vi "NetworkPlots.vi"(10 "ControlRefs":T1, 11 "VisualizeData":T2 {"clPmuImpairRptArray"."Synx" format="%#_4g"; "clEvtReportArray"."Synx" format="%#_4g"}) -> ()   [LabVIEW 2014, in "Visualization.lvlib" / "VisualizeNetwork_class.lvclass"]
uses:
  VisualizeNetwork_class.lvclass
  VisializeBase_class/Typedefs/VisualizeData.ctl
  VisializeBase_class/Typedefs/clVisualizeData.ctl
  Modules/EventPlugins/EventPluginBaseClass/TypeDefs/clEvtReportArray.ctl
  Modules/EventPlugins/EventPluginBaseClass/TypeDefs/clEvtReport.ctl
  Modules/EventPlugins/EventPluginBaseClass/TypeDefs/dblEvtSignalArray.ctl
  Modules/NetworkImpairmentModule/PublicAPI/Arguments/Broadcasts/dblNetworkTime.ctl
  Modules/NetworkImpairmentModule/PublicAPI/Arguments/Broadcasts/dblPktLoss.ctl
  Modules/FlagImpairModule/PublicAPI/Arguments/Broadcasts/ui32FlagImpairmentArray.ctl
  Modules/EventPlugins/EventPluginBaseClass/EventPluginBaseClass.lvclass
  Modules/NetworkImpairmentModule/NetworkImpairmentModule.lvlib
  Modules/FlagImpairModule/FlagImpairModule.lvlib
  VisializeBase_class/VisualizeBase_class.lvclass
  VisualizeApp_class/VisualizeAppBase_class.lvclass
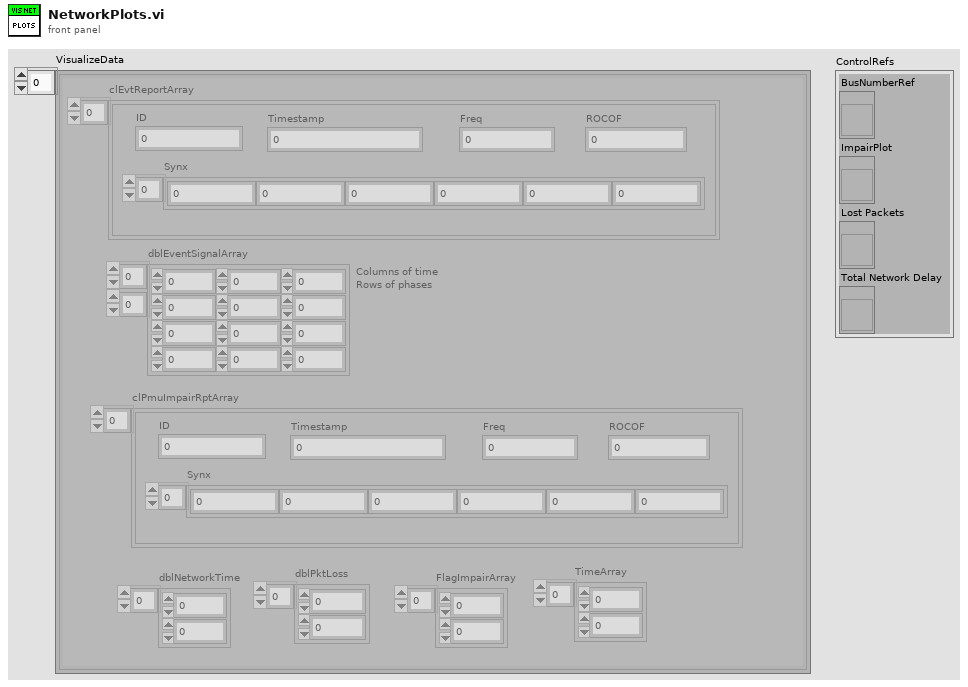
[diagram p1: front panel]
types:
  T1 = cluster{"BusNumberRef":refnum<vi>, "ImpairPlot":refnum<vi>, "Lost Packets":refnum<vi>, "Total Network Delay":refnum<vi>}
  T2 = typedef "Visualization.lvlib/VisualizeBase_class.lvclass/VisualizeData.ctl" = T3[]
  T3 = typedef "Visualization.lvlib/VisualizeAppBase_class.lvclass/clVisualizeData.ctl" = cluster{"clEvtReportArray":T4, "dblEventSignalArray":T6, "clPmuImpairRptArray":T4, "dblNetworkTime":T7, "dblPktLoss":T8, "FlagImpairArray":T9, "TimeArray":dbl[]}
  T4 = typedef "EventPlugins.lvlib/EventPluginBaseClass.lvclass/clEvtReportArray.ctl" = T5[]
  T5 = typedef "EventPlugins.lvlib/EventPluginBaseClass.lvclass/clEvtReport.ctl" = cluster{"Timestamp":dbl, "Synx":cdb[], "Freq":dbl, "ROCOF":dbl, "ID":i16}
  T6 = typedef "EventPlugins.lvlib/EventPluginBaseClass.lvclass/dblEvtSignalArray.ctl" = dbl[][]
  T7 = typedef "NetworkImpairmentModule.lvlib/dblNetworkTime.ctl" = dbl[]
  T8 = typedef "NetworkImpairmentModule.lvlib/dblPktLoss.ctl" = dbl[]
  T9 = typedef "FlagImpairModule.lvlib/ui32FlagImpairmentArray.ctl" = u32[]
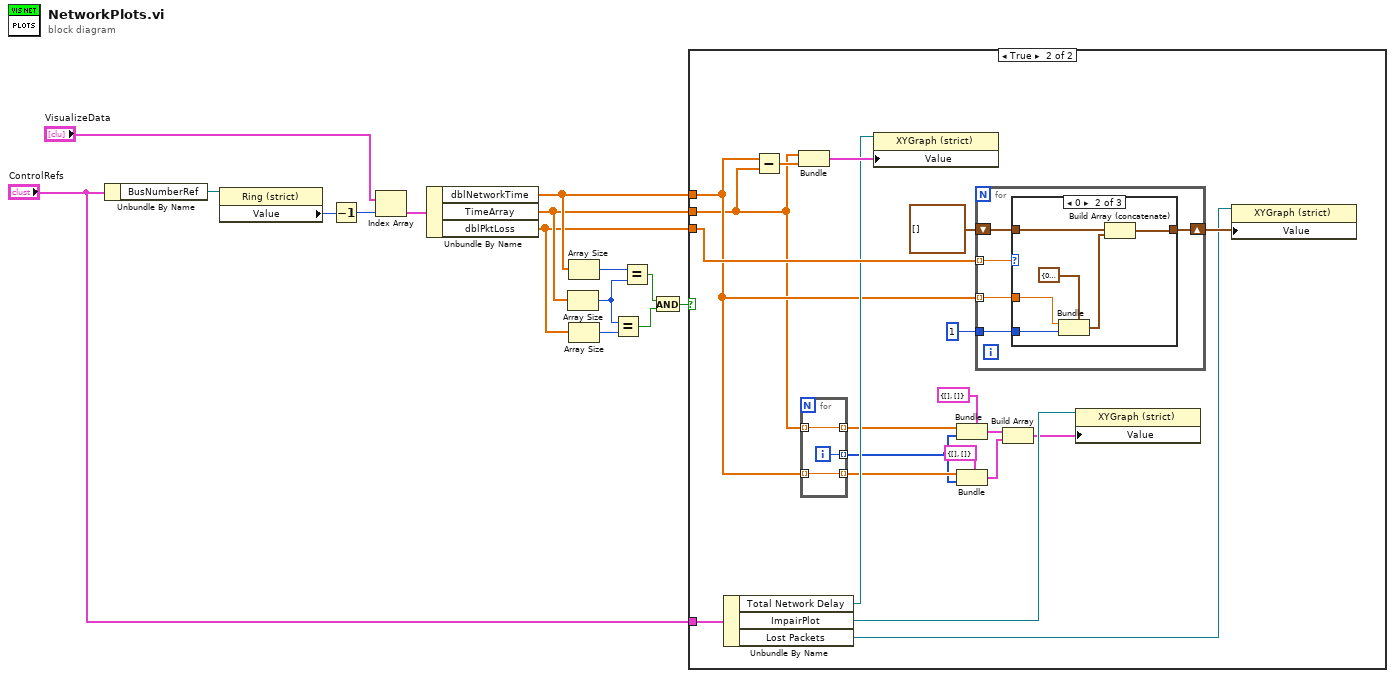
[diagram p0: block diagram]
diagram:
  n1 = Unbundle By Name("ControlRefs") -> ("BusNumberRef"=w15:refnum<vi>)
  n2 = property class="Ring (strict)"(reference=w15) -> ("Value"=w14:u8)  [unwired: 1 in, 2 out]
  n3 = Decrement(x=w14) -> (x-1=w13:u8)
  n4 = Index Array(array="VisualizeData", index=w13) -> (element=w11:T3)
  n5 = Unbundle By Name(w11) -> ("dblNetworkTime"=w4:T7, "TimeArray"=w3:dbl[], "dblPktLoss"=w2:T8)
  n6 = Array Size(array=w3) -> (size(s)=w8:i32)
  n7 = Array Size(array=w4) -> (size(s)=w9:i32)
  n8 = Array Size(array=w2) -> (size(s)=w10:i32)
  n9 = Equal?(x=w8, y=w10) -> (x = y?=w6:bool)
  n10 = Equal?(x=w9, y=w8) -> (x = y?=w7:bool)
  n11 = And(x=w7, y=w6) -> (x .and. y?=w1:bool)
  n12 = case shown="True" w1 {
    tunnel: "ControlRefs" -> [_ w35]
    tunnel: w4 -> [_ w19]
    tunnel: w3 -> [_ w17]
    tunnel: w2 -> [_ w31]
    frame False {
    }
    frame True {
      n13 = Unbundle By Name(w35) -> ("Total Network Delay"=w28:refnum<vi>, "ImpairPlot"=w24:refnum<vi>, "Lost Packets"=w25:refnum<vi>)
      n14 = Subtract(x=w19, y=w17) -> (x-y=w34:T7)
      n15 = Bundle("TimeArray"=w17, "dblNetworkTime"=w34) -> (w33:cluster{"TimeArray":dbl[], "dblNetworkTime":T7})  [unwired: 1 in]
      n16 = for {
        tunnel: w19 -> [w38] mode=indexing
        tunnel: [w38] -> w20 mode=indexing
        tunnel: [w37] -> w16 mode=indexing
        tunnel: w17 -> [w36] mode=indexing
        tunnel: [w36] -> w18 mode=indexing
        i -> [w37]
      }
      n17 = property class="XYGraph (strict)"(reference=w28, "Value"=w33) -> ()  [unwired: 1 in, 2 out]
      n18 = Bundle(cluster=cluster{dbl[], i32[]} {[], []}, w18, w16) -> (w27:cluster{dbl[], i32[]})
      n19 = Bundle(cluster=cluster{dbl[], i32[]} {[], []}, w20, w16) -> (w26:cluster{dbl[], i32[]})
      n20 = for {
        tunnel: w31 -> [w43] mode=indexing
        shift-right: [w41] -> w29
        shift-left: cluster{"NetworkTime":dbl, "BusIndex":u16}[] [] -> [w42]
        tunnel: w19 -> [w40] mode=indexing
        tunnel: u16 1 ("BusIndex") -> [w39]
        n21 = case shown="0" w43 {
          tunnel: w42 -> [_ w49 w50]
          tunnel: [_ w47 w50] -> w41
          tunnel: w40 -> [_ w46 _]
          tunnel: w39 -> [_ w44 _]
          frame Default {
          }
          frame 0 {
            n22 = Bundle(cluster=cluster{"NetworkTime":dbl, "BusIndex":u16} {"NetworkTime"=0.0, "BusIndex"=0}, "NetworkTime"=w46, "BusIndex"=w44) -> (w48:cluster{"NetworkTime":dbl, "BusIndex":u16})
            n23 = Build Array (concatenate)(w49, w48) -> (w47:cluster{"NetworkTime":dbl, "BusIndex":u16}[])
          }
          frame 1 {
          }
        }
      }
      n24 = Build Array(w27, w26) -> (w23:cluster{dbl[], i32[]}[])
      n25 = property class="XYGraph (strict)"(reference=w24, "Value"=w23) -> ()  [unwired: 1 in, 2 out]
      n26 = property class="XYGraph (strict)"(reference=w25, "Value"=w29) -> ()  [unwired: 1 in, 2 out]
    }
  }
